vi "Operation Complete.vi"(8 "error in (no error)":errorcluster, 11 "Session In":refnum<visa-resource-name>) -> (0 "error out":errorcluster, 2 "Operation Complete":bool, 3 "Session Out":refnum<visa-resource-name>)   [LabVIEW 2023, in "HAF.lvlib" / "Driver.lvclass"]
doc: "Checks to see if any existing operations being executed on an instrument have finished."
uses:
  Driver.lvclass
  Driver.lvclass/Driver.ctl
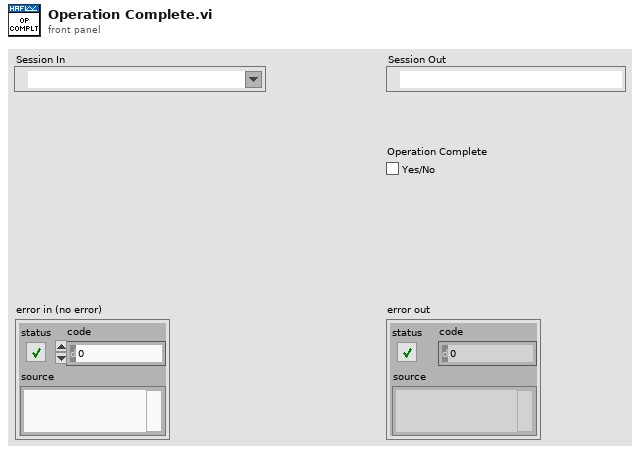
[diagram p1: front panel]
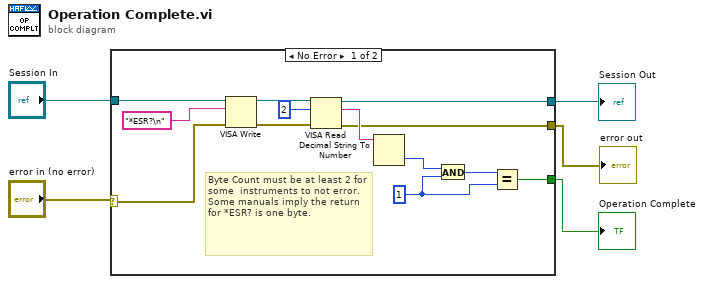
[diagram p0: block diagram]
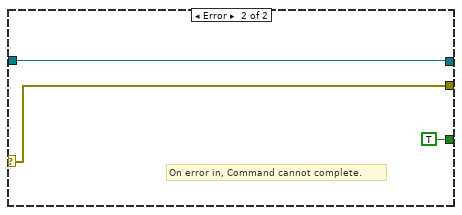
[diagram p2: hidden frame]
diagram:
  n1 = case shown="No Error" "error in (no error)" {
    selector: "error in (no error)" -> [w16 w20]
    tunnel: "Session In" -> [w18 w19]
    tunnel: [w8 TRUE] -> w1
    tunnel: [w7 w20] -> w2
    tunnel: [w6 w19] -> w3
    frame No Error {
      w9 = 1 ("y")
      # "Byte Count must be at least 2 for some  instruments to not error.  Some manuals imply the return for *ESR? is one byte."
      n2 = VISA Write(VISA resource name=w18, write buffer="*ESR?\n", error in (no error)=w16) -> (VISA resource name out=w15:refnum<visa-resource-name>, error out=w14:errorcluster)  [unwired: 1 out]
      n3 = VISA Read(VISA resource name=w15, byte count=u32 2, error in (no error)=w14) -> (VISA resource name out=w6:refnum<visa-resource-name>, read buffer=w12:string, error out=w7:errorcluster)  [unwired: 1 out]
      n4 = Decimal String To Number(string=w12) -> (number=w11:i32)  [unwired: 2 in, 1 out]
      n5 = And(x=w11, y=w9) -> (x .and. y?=w10:i32)
      n6 = Equal?(x=w10, y=w9) -> (x = y?=w8:bool)
    }
    frame Error {
      # "On error in, Command cannot complete."
    }
  }
  "Operation Complete" <- w1
  "Session Out" <- w3
  "error out" <- w2
